vi "Smart Open.vi"(7 "Allow multiple opens?":bool=TRUE, 8 "error in (no error)":errorcluster, 10 "Channel Names":tag[](array[tag])) -> (0 "error out":errorcluster, 3 "DO (N Samples) Ref Out":T1)   [LabVIEW 2021, in "DO Block.lvlib"]
doc: "Opens the reference to the digital output block write channel (ConnectorA/DIO1). You must open a reference before you write values."
uses:
  <vilib>/myRIO/Instrument Drivers/Onboard IO/DO Block/DO Block.lvlib
  <vilib>/myRIO/Common/Instrument Driver Framework/Utilities/typedefs/Hardware Version Enum.ctl
  <vilib>/myRIO/Common/Instrument Driver Framework/Utilities/typedefs/Generic FPGA Reference.ctl
  <vilib>/myRIO/Common/Instrument Driver Framework/Utilities/typedefs/myRIO v1.0 Reference.ctl
  <vilib>/myRIO/Common/Instrument Driver Framework/Utilities/typedefs/myRIO Generic Hardware Reference.ctl
  <vilib>/myRIO/Common/Instrument Driver Framework/myRIO v1.0/DO Block/typedefs/DO Block Channels Enum.ctl
  <vilib>/myRIO/Common/Instrument Driver Framework/myRIO v1.0/DO Block/typedefs/DO Block Channels List.ctl
  <vilib>/myRIO/Instrument Drivers/Onboard IO/DO Block/typedefs/DO Block Reference.ctl
  <vilib>/myRIO/Instrument Drivers/Onboard IO/DO Block/vis/myRIO DO N Samples Open.xnode
  <vilib>/myRIO/Common/Instrument Driver Framework/myRIO v1.0/DO Block/vis/myRIO v1.1 Open Throughput DO (N Samples).vi
  <vilib>/userdefined/High Color/nirio_resource_hc.ctl
  <vilib>/myRIO/Instrument Drivers/Utilities/Utilities.lvlib
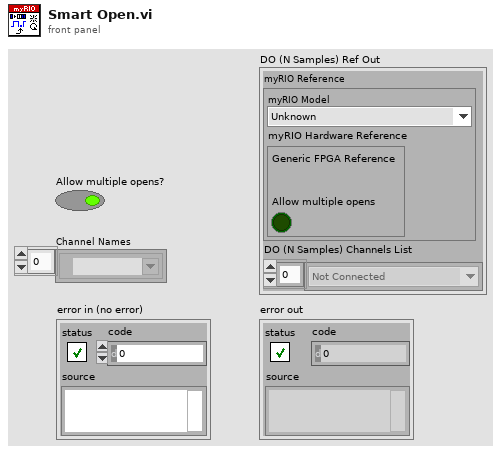
[diagram p1: front panel]
types:
  T1 = typedef "DO Block.lvlib/DO Block Reference.ctl" = cluster{"myRIO Reference":T2, "DO (N Samples) Channels List":T6}
  T2 = typedef "myRIO Generic Hardware Reference.ctl" = cluster{"myRIO Model":T3, "myRIO Hardware Reference":T4}
  T3 = typedef "Hardware Version Enum.ctl" = enum16{"Unknown", "myRIO-1900", "myRIO-1950", "roboRIO", "NI ELVIS RIO CM", "ELVIS III"}
  T4 = typedef "myRIO v1.0 Reference.ctl" = cluster{"Generic FPGA Reference":T5, "Allow multiple opens":bool}
  T5 = typedef "Generic FPGA Reference.ctl" = refnum<k20>
  T6 = typedef "DO Block Channels List.ctl" = T7[]
  T7 = typedef "DO Block Channels Enum.ctl" = enum16{"Not Connected", "A/DO0 (N Samples)", "A/DO1 (N Samples)", "A/DO2 (N Samples)", "A/DO3 (N Samples)", "A/DO4 (N Samples)", "A/DO5 (N Samples)", "A/DO6 (N Samples)", "A/DO7 (N Samples)", "A/DO8 (N Samples)", "A/DO9 (N Samples)", "A/DO10 (N Samples)", "A/DO11 (N Samples)", "A/DO12 (N Samples)", "A/DO13 (N Samples)", "A/DO14 (N Samples)", "A/DO15 (N Samples)", "A/DO16 (N Samples)", "A/DO17 (N Samples)", "A/DO18 (N Samples)", "A/DO19 (N Samples)", "B/DO0 (N Samples)", "B/DO1 (N Samples)", "B/DO2 (N Samples)", "B/DO3 (N Samples)", "B/DO4 (N Samples)", "B/DO5 (N Samples)", "B/DO6 (N Samples)", "B/DO7 (N Samples)", "B/DO8 (N Samples)", "B/DO9 (N Samples)", "B/DO10 (N Samples)", "B/DO11 (N Samples)", "B/DO12 (N Samples)", "B/DO13 (N Samples)", "B/DO14 (N Samples)", "B/DO15 (N Samples)", "B/DO16 (N Samples)", "B/DO17 (N Samples)", "B/DO18 (N Samples)", "B/DO19 (N Samples)"}
  T8 = typedef "nirio_resource_hc.ctl" = tag
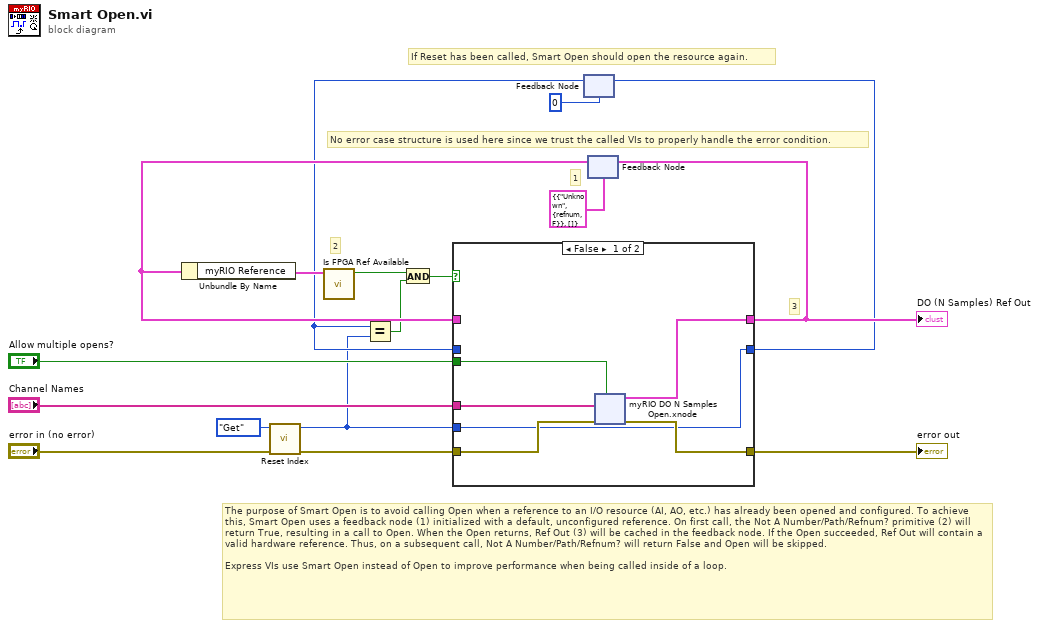
[diagram p0: block diagram]
diagram:
  # "If Reset has been called, Smart Open should open the resource again."
  # "No error case structure is used here since we trust the called VIs to properly handle the error condition."
  # "3"
  # "1"
  # "2"
  # "The purpose of Smart Open is to avoid calling Open when a reference to an I/O resource (AI, AO, etc.) has already been opened and configured. To achieve this, Smart Open uses a feedback node (1) initialized with a default, unconfigured reference. On first call, the Not A Number/Path/Refnum? primitive (2) will return True, resulting in a call to Open. When the Open returns, Ref Out (3) will be cached in the feedback node. If the Open succeeded, Ref Out will contain a valid hardware reference. Thus, on a subsequent call, Not A Number/Path/Refnum? will return False and Open will be skipped.\n\t\nExpress VIs use Smart Open instead of Open to improve performance when being called inside of a loop."
  n1 = call <vilib>:"Reset Index.vi"("error in (no error)"="error in (no error)", "Action"=enum16{"Get", "Set"}."Get") -> ("error out"=w7:errorcluster, "Ref Count"=w2:u8)  [unwired: 8 in]
  n2 = feedback #1(u8 0 ("Ref Count")) -> (w6:u8)
  n3 = Equal?(x=w6, y=w2) -> (x = y?=w4:bool)
  n4 = feedback #2(T1 {"myRIO Reference"={"myRIO Model"=enum."Unknown", "myRIO Hardware Reference"={"Generic FPGA Reference"=refnum, "Allow multiple opens"=FALSE}}, "DO (N Samples) Channels List"=[]} ("DO (N Samples) Write Ref Out")) -> (w17:T1)
  n5 = Unbundle By Name(w17) -> ("myRIO Reference"=w11:T2)
  n6 = call <vilib>:"Is FPGA Ref Available.vi"("myRIO Reference"=w11) -> ("Is Available?"=w5:bool)  [unwired: 10 in]
  n7 = And(x=w5, y=w4) -> (x .and. y?=w3:bool)
  n8 = case shown="False" w3 {
    tunnel: w7 -> [w23 w41]
    tunnel: [w22 w42] -> w13
    tunnel: [w21 w41] -> w16
    tunnel: w17 -> [_ w42]
    tunnel: "Channel Names" -> [w20 _]
    tunnel: "Allow multiple opens?" -> [w19 _]
    tunnel: [w18 w40] -> w9
    tunnel: w6 -> [_ w40]
    tunnel: w2 -> [w18 _]
    frame False {
      n9 = xnode "myRIO DO N Samples Open.xnode"("error in (no error)"=w23, "Allow multiple opens?"=w19, "Channel Names"=w20) -> ("error out"=w21:errorcluster, "DO (N Samples) Ref Out"=w22:T1)
    }
    frame True {
    }
  }
  "DO (N Samples) Ref Out" <- w13
  "error out" <- w16
  n10 = feedback-in #1(w9) -> ()
  n11 = feedback-in #2(w13) -> ()
